vi "Read Parent Attributes.vi"(11 "TEMPLATE Actor in":refnum<class "TEMPLATE Actor.lvclass">) -> (2 "Parent Attributes":refnum<class "Attributes.lvclass">)   [LabVIEW 2025, in "_Template.lvlib" / "Templates.lvlib" / "TEMPLATE Actor.lvlib" / "TEMPLATE Actor.lvclass"]
uses:
  TEMPLATE Actor.lvclass
  jettl/jettl/Attributes/Attributes/Attributes.lvclass
  TEMPLATE Actor.lvclass/TEMPLATE Actor.ctl
  jettl/jettl/Actor/Actor/Actor.lvclass
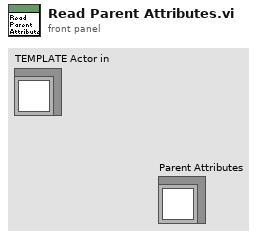
[diagram p1: front panel]
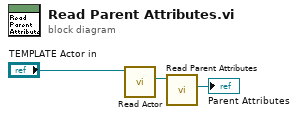
[diagram p0: block diagram]
diagram:
  n1 = call-dynamic "Read Actor.vi"("TEMPLATE Actor in"="TEMPLATE Actor in") -> ("Actor"=w1:refnum<class "Actor.lvclass">)  [unwired: 10 in]
  n2 = call-dynamic "Read Parent Attributes.vi"("Actor in"=w1) -> ("Parent Attributes"=→"Parent Attributes":refnum<class "Attributes.lvclass">)  [unwired: 10 in]
